vi "Abort.vi"(8 "error in (no error)":errorcluster, 11 "SMO":refnum<class "SMO.lvclass">) -> (0 "error out":errorcluster, 3 "SMO out":refnum<class "SMO.lvclass">)   [LabVIEW 2013, in "SMO.lvclass"]
doc: "---------------------------------------------------------------\nJKI State Machine Objects™\nhttp://jki.net/state-machine-objects/\nCopyright (C) 2005-2015, JKI <info@jki.net>\nALL RIGHTS RESERVED"
uses:
  SMO.lvclass
  SMO.lvclass/SMO.ctl
panel:
  # "For instructions on how to use the JKI State Machine Objects, examples and video tutorials, visit:\nhttp://jki.net/state-machine-objects/\n\nJKI State Machine Objects™\nhttp://jki.net/state-machine-objects/\nCopyright (C) 2005-2015, JKI <info@jki.net>\nALL RIGHTS RESERVED"
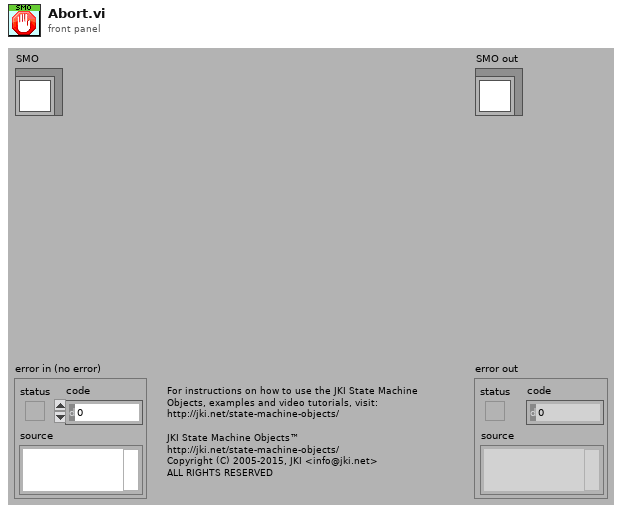
[diagram p1: front panel]
types:
  T1 = typedef "SMO.lvclass/PrivateData--Ref.ctl" = refnum<data-value>
  T2 = typedef "SMO.lvclass/PrivateData--Cluster.ctl" = cluster{"Parent Call":T3, "Registered Processes":T4[], "Sync Notifier":refnum<notifier>, "Process Error Notifier":refnum<notifier>, "Protected Events":T5, "Public Events":T6, "SMO State":T7, "[Dependencies]":T8[], "[Attributes]":refnum<class "Attribute.lvclass">[], "Launcher Close":refnum<notifier>, "Caller Watchdog":refnum<queue>, "Accessibility":T9}
  T3 = typedef "SMO.lvclass/Parent Call--Enum.ctl" = enum16{"Allows parent to run", "Does not request parent to run"}
  T4 = typedef "SMO.lvclass/RegisteredProcessData--Cluster.ctl" = cluster{"Name":string, "Static VI Ref":refnum<vi>, "Running":bool, "NotifierRef":u32}
  T5 = typedef "SMO.lvclass/Protected Events.ctl" = cluster{"StopProcesses":refnum<user-event>, "AbortProcesses":refnum<user-event>, "Config Changed":refnum<user-event>, "Dependency":refnum<user-event>}
  T6 = typedef "SMO.lvclass/Public Events.ctl" = cluster{"Error":refnum<user-event>, "State":refnum<user-event>, "Reserve State":refnum<user-event>}
  T7 = typedef "SMO.lvclass/SMOState --Enum.ctl" = enum16{"unknown", "Created", "Started", "Stopped"}
  T8 = typedef "SMO.lvclass/SMO Dependency--Cluster.ctl" = cluster{"Dependency":refnum<class "SMO.lvclass">, "Level":string}
  T9 = typedef "SMO.lvclass/Accessibility--Cluster.ctl" = cluster{"Lock Key":string, "Reserve State":T10}
  T10 = typedef "SMO.lvclass/Reserve State--Enum.ctl" = enum16{"Unreserved", "Reserved", "Self-locked"}
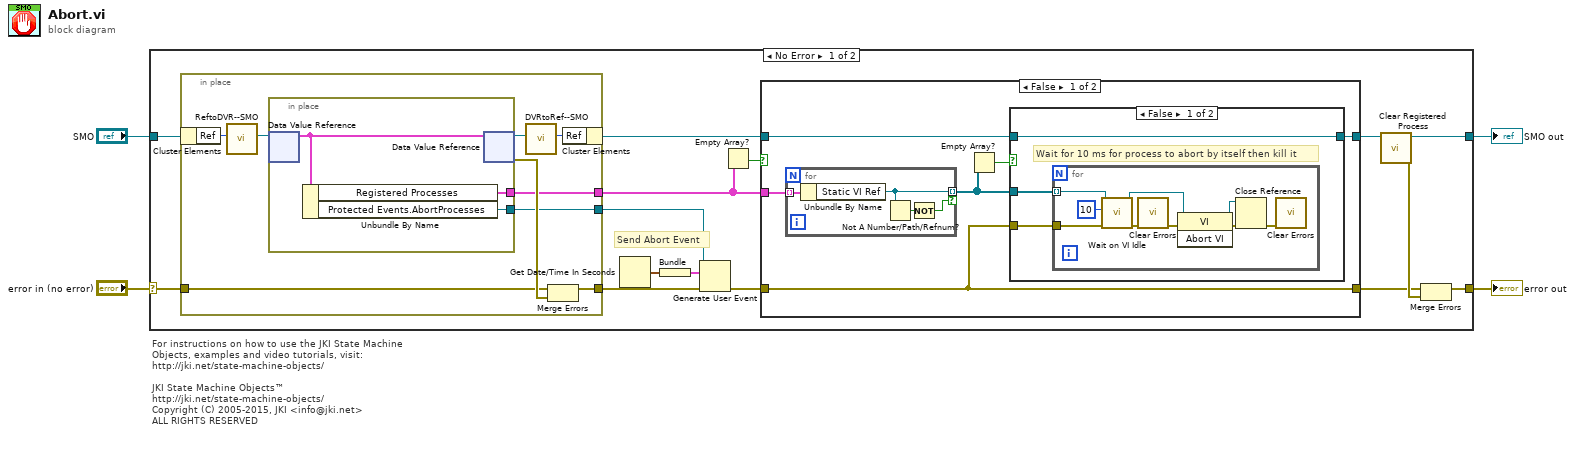
[diagram p0: block diagram]
diagram:
  # "For instructions on how to use the JKI State Machine Objects, examples and video tutorials, visit:\nhttp://jki.net/state-machine-objects/\n\nJKI State Machine Objects™\nhttp://jki.net/state-machine-objects/\nCopyright (C) 2005-2015, JKI <info@jki.net>\nALL RIGHTS RESERVED"
  n1 = case shown="No Error" "error in (no error)" {
    selector: "error in (no error)" -> [w18 w58]
    tunnel: [w13 w58] -> w3
    tunnel: [w12 w57] -> w1
    tunnel: "SMO" -> [w19 w57]
    frame No Error {
      # "Send Abort Event"
      n2 = in-place {
        in-place-border: w18 -> [w49]
        in-place-border: [w52] -> w14
        in-place-border: [w51] -> w15
        in-place-border: [w50] -> w8
        n3 = in-place-cluster #1(w19) -> ("Ref"=w48:u32)
        n4 = call "ReftoDVR--SMO.vi"("Ref"=w48) -> ("Ref"=w47:T1)  [unwired: 10 in]
        n5 = in-place {
          in-place-border: [w54] -> w51
          in-place-border: [w55] -> w50
          n6 = in-place-dvr #2(w47) -> (w56:T2)  [unwired: 1 out]
          n7 = Unbundle By Name(w56) -> ("Registered Processes"=w55:T4[], "Protected Events.AbortProcesses"=w54:refnum<user-event>)
          n8 = in-place-dvr #2(w56) -> (w46:T1, w53:errorcluster)
        }
        n9 = call "DVRtoRef--SMO.vi"("Ref"=w46) -> ("Ref"=w45:u32)  [unwired: 10 in]
        n10 = Merge Errors(w49, w53) -> (w52:errorcluster)
        n11 = in-place-cluster #1("Ref"=w45) -> (w7:refnum<class "SMO.lvclass">)
      }
      n12 = Get Date/Time In Seconds() -> (seconds since 1Jan1904=w16:timestamp)
      n13 = Bundle("seconds since 1Jan1904"=w16) -> (w17:cluster{"seconds since 1Jan1904":timestamp})  [unwired: 1 in]
      n14 = Generate User Event(user event=w15, event data cluster=w17, error in=w14) -> (error out=w10:errorcluster)  [unwired: 1 in, 1 out]
      n15 = Empty Array?(array=w8) -> (empty?=w9:bool)
      n16 = case shown="False" w9 {
        tunnel: w8 -> [w25 _]
        tunnel: w10 -> [w24 w43]
        tunnel: w7 -> [w22 w44]
        tunnel: [w21 w44] -> w6
        tunnel: [w24 w43] -> w5
        frame False {
          n17 = for {
            tunnel: w25 -> [w40] mode=indexing
            tunnel: [w39] -> w23 mode=indexing if=w41
            n18 = Unbundle By Name(w40) -> ("Static VI Ref"=w39:refnum<vi>)
            n19 = Not A Number/Path/Refnum?(number/path/refnum=w39) -> (NaN/Path/Refnum?=w42:bool)
            n20 = Not(x=w42) -> (.not. x?=w41:bool)
          }
          n21 = Empty Array?(array=w23) -> (empty?=w20:bool)
          n22 = case shown="False" w20 {
            tunnel: w24 -> [w28 _]
            tunnel: w23 -> [w27 _]
            tunnel: w22 -> [w26 w38]
            tunnel: [w26 w38] -> w21
            frame False {
              # "Wait for 10 ms for process to abort by itself then kill it"
              n23 = for {
                tunnel: w28 -> [w37]
                tunnel: w27 -> [w29] mode=indexing
                n24 = call "Wait on VI Idle.vi"("error in (no error)"=w37, "ms Timout (100ms)"=u32 10, "VI to Wait on"=w29) -> ("error out"=w35:errorcluster, "VI to Wait on dup"=w30:refnum<vi>)  [unwired: 6 in, 1 out]
                n25 = call <vilib>:"Clear Errors.vi"("error in (no error)"=w35) -> ("error out"=w34:errorcluster)  [unwired: 6 in]
                n26 = invoke class="VI" method="Abort VI"(reference=w30, error in=w34) -> (reference out=w31:refnum<vi>, error out=w33:errorcluster)  [unwired: 1 in, 1 out]
                n27 = Close Reference(reference=w31, error in (no error)=w33) -> (error out=w32:errorcluster)
                n28 = call <vilib>:"Clear Errors.vi"("error in (no error)"=w32) -> ()  [unwired: 6 in, 1 out]
              }
            }
            frame True {
            }
          }
        }
        frame True {
        }
      }
      n29 = call "Clear Registered Process.vi"("SMO"=w6) -> ("error out"=w11:errorcluster, "SMO out"=w12:refnum<class "SMO.lvclass">)  [unwired: 9 in]
      n30 = Merge Errors(w5, w11) -> (w13:errorcluster)
    }
    frame Error {
    }
  }
  "error out" <- w3
  "SMO out" <- w1
